vi "SSC DCPower Expanded Pin List to SSC Index.vi"(0 "DCPower SSC In":T1[](array[typedef]), 5 "Expanded Pin Information":T2[](array[typedef])) -> (4 "Indexes Out":i32[](array[numeric]))   [LabVIEW 2020]
uses:
  Shared SubVIs/TSM Pin Abstraction/TSM Expanded Pin Information.ctl
  Shared SubVIs/TSM Pin Abstraction/TSM Pin Type Identifier.ctl
  SSC DCPower/SSC DCPower.ctl
  Shared SubVIs/Trim Whitespace [Inlined].vi
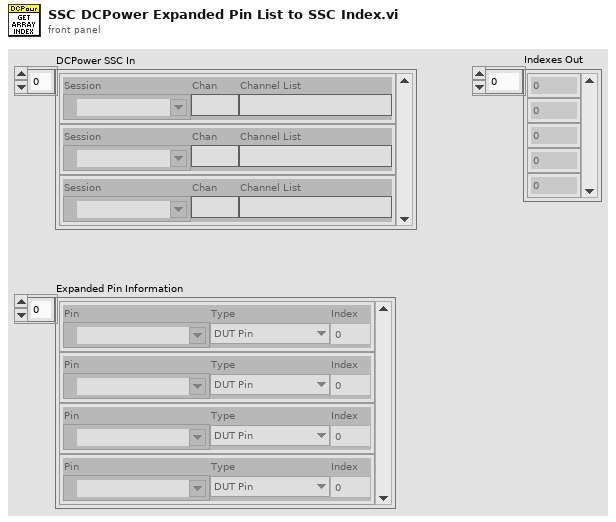
[diagram p1: front panel]
types:
  T1 = typedef "SSC DCPower.ctl" = cluster{"Session":refnum<k15>, "Chan":string, "Channel List":string}
  T2 = typedef "TSM Expanded Pin Information.ctl" = cluster{"Pin":tag, "Type":T3, "Index":i32}
  T3 = typedef "TSM Pin Type Identifier.ctl" = enum8{"DUT Pin", "System Pin", "Pin Group", "Not Determined"}
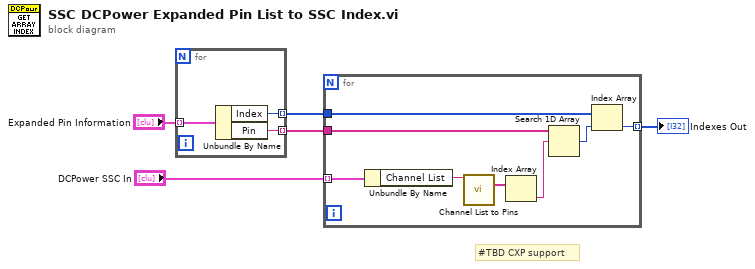
[diagram p0: block diagram]
diagram:
  # "#TBD CXP support"
  n1 = for {
    tunnel: "Expanded Pin Information" -> [w8] mode=indexing
    tunnel: [w7] -> w3 mode=indexing
    tunnel: [w6] -> w2 mode=indexing
    n2 = Unbundle By Name(w8) -> ("Index"=w6:i32, "Pin"=w7:tag)
  }
  n3 = for {
    tunnel: "DCPower SSC In" -> [w16] mode=indexing
    tunnel: w3 -> [w13]
    tunnel: w2 -> [w11]
    tunnel: [w9] -> w1 mode=indexing
    n4 = Unbundle By Name(w16) -> ("Channel List"=w15:string)
    n5 = call "Channel List to Pins.vi"("Channel List"=w15) -> ("Pins"=w14:tag[])  [unwired: 12 in, 2 out]
    n6 = Index Array(array=w14) -> (element=w12:tag)  [unwired: 1 in]
    n7 = Search 1D Array(1D array=w13, element=w12) -> (index of element=w10:i32)  [unwired: 1 in]
    n8 = Index Array(array=w11, index=w10) -> (element=w9:i32)
  }
  "Indexes Out" <- w1
